vi "SimpleError.vi"(8 "error in (no error)":errorcluster, 11 "map":map{string, string}(c390)) -> (0 "error out":errorcluster, 2 "status":string="error", 3 "description":string)   [LabVIEW 2021]
uses:
  b9720b65-f77a-49f2-89bf-c9170129f96c.vi
  <vilib>/JDP Science/JSONtext/Next JSON Value.vi
  <vilib>/JDP Science/JSONtext/String Subset.vi
  <vilib>/JDP Science/JSONtext/Parsing/Advance past next JSON Value (inlined COPY).vi
  <vilib>/JDP Science/JSONtext/Parsing/Advance past whitespace.vi
  <vilib>/JDP Science/JSONtext/Parsing/Advance past String.vi
  <vilib>/JDP Science/JSONtext/Parsing/Advance past Number.vi
  <vilib>/JDP Science/JSONtext/Parsing/Advance past Line Ending.vi
  <vilib>/JDP Science/JSONtext/Parsing/Parse Full Path or Item Name.vi
  <vilib>/JDP Science/JSONtext/Parsing/Advance past Array.vi
  <vilib>/JDP Science/JSONtext/Parsing/Advance past Object.vi
  <vilib>/JDP Science/JSONtext/support/Error Cluster From Code.vi
  <vilib>/JDP Science/JSONtext/Offset/Find Item Locations by Path.vi
  <vilib>/JDP Science/JSONtext/JSON text to Variant.vi
  <vilib>/JDP Science/JSONtext/LVClass Serializer/JSONtext LVClass Serializer.lvclass
  <vilib>/JDP Science/JSONtext/JSONtext.lvlib
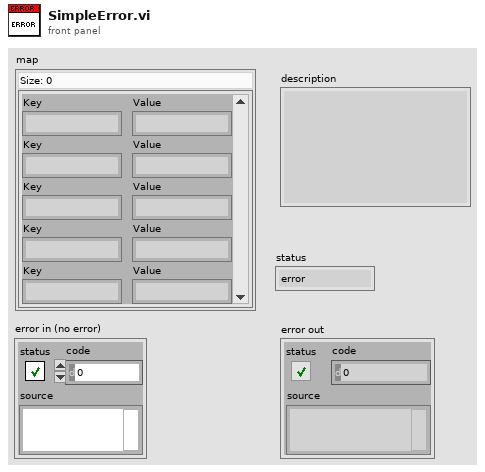
[diagram p1: front panel]
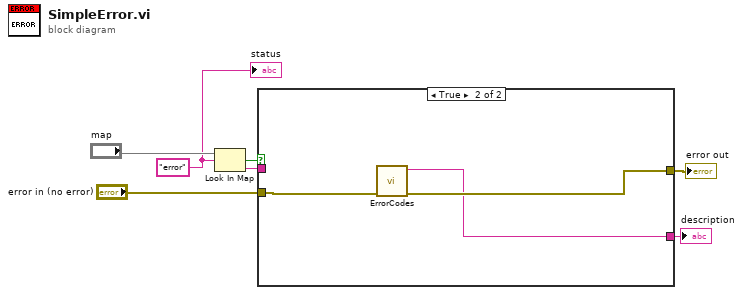
[diagram p0: block diagram]
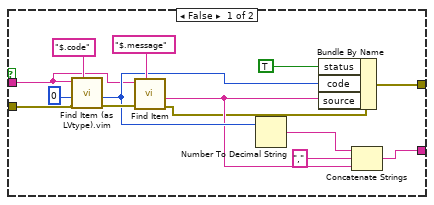
[diagram p2: hidden frame]
diagram:
  w6 = "error" ("key")
  n1 = Look In Map(map="map", key=w6) -> (key not found?=w5:bool, value=w4:string)  [unwired: 1 in]
  n2 = case shown="True" w5 {
    tunnel: w4 -> [w10 _]
    tunnel: "error in (no error)" -> [w19 w24]
    tunnel: [w8 w23] -> w3
    tunnel: [w11 w22] -> w2
    frame False {
      n3 = call "Find Item (as LVtype).vim"("$Path or Item Name"="$.code", "error in (no error)"=w19, "Data Type and Default Value"=0, "JSON"=w10) -> ("error out"=w18:errorcluster, "Data"=w15:i32)  [unwired: 4 in, 2 out]
      n4 = call <vilib>:"Find Item.vi"("$Path or Item Name"="$.message", "error in (no error)"=w18, "JSON"=w10) -> ("error out"=w9:errorcluster, "<JSON>"=w13:string)  [unwired: 5 in, 2 out]
      n5 = Number To Decimal String(number=w15) -> (decimal integer string=w14:string)  [unwired: 1 in]
      n6 = Bundle By Name(cluster=w9, "status"=TRUE, "code"=w15, "source"=w13) -> (w8:errorcluster)
      n7 = Concatenate Strings(w14, "," ("string"), w13) -> (w11:string)
    }
    frame True {
      n8 = call "ErrorCodes.vi"("error in (no error)"=w24) -> ("error out"=w23:errorcluster, "description"=w22:string)  [unwired: 9 in]
    }
  }
  "error out" <- w3
  "description" <- w2
  "status" <- w6
